vi "AB_Engine_CreateMissingVIsTree.vi"(10 "All VIs":T1[](array[typedef]), 11 "Missing VIs":T1[](array[typedef])) -> (3 "Missing VIs tree":variant)   [LabVIEW 2020]
uses:
  <vilib>/AppBuilder/Engine/AB_Engine_PathNode.ctl
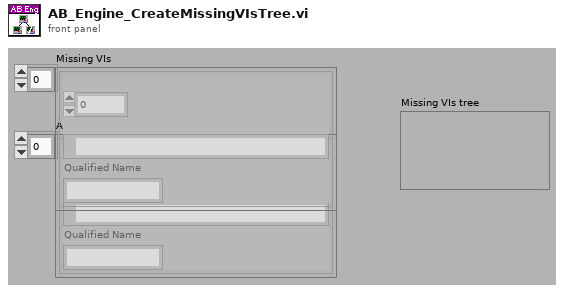
[diagram p1: front panel]
types:
  T1 = typedef "AB_Engine_PathNode.ctl" = cluster{"parent":i32, "path":path, "Qualified Name":string}
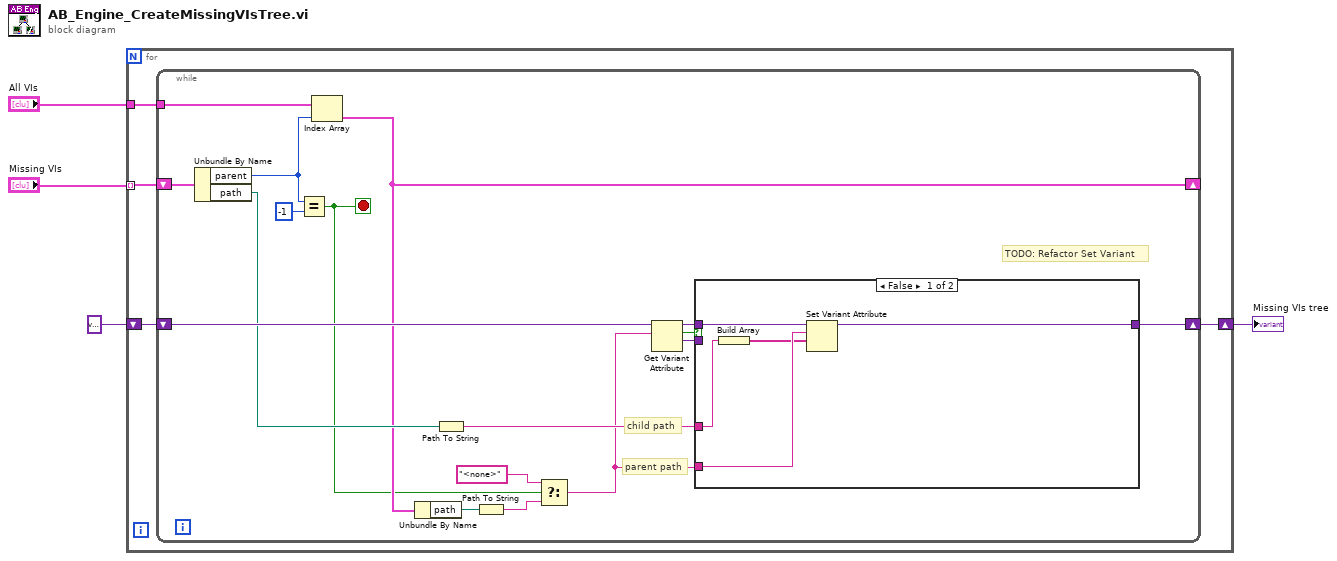
[diagram p0: block diagram]
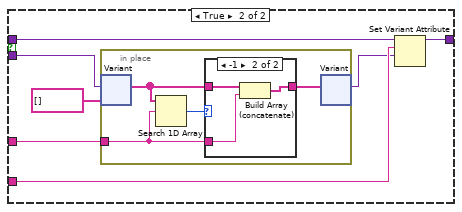
[diagram p2: hidden frame]
diagram:
  n1 = for {
    tunnel: "Missing VIs" -> [w7] mode=indexing
    tunnel: "All VIs" -> [w8]
    shift-right: [w5] -> w1
    shift-left: variant ("Node indices") -> [w6]
    n2 = while {
      tunnel: w8 -> [w25]
      shift-right: [w18] -> _
      shift-left: w7 -> [w20]
      shift-right: [w21] -> w5
      shift-left: w6 -> [w22]
      stop <- w11 stop-if-true
      # "TODO: Refactor Set Variant"
      # "parent path"
      # "child path"
      n3 = Unbundle By Name(w20) -> ("parent"=w24:i32, "path"=w19:path)
      n4 = Equal?(x=w24, y=-1) -> (x = y?=w11:bool)
      n5 = Index Array(array=w25, index=w24) -> (element=w18:T1)
      n6 = Unbundle By Name(w18) -> ("path"=w13:path)
      n7 = Path To String(path=w19) -> (string=w14:string)
      n8 = Path To String(path=w13) -> (string=w10:string)
      n9 = Select(t="<none>" ("f"), s=w11, f=w10) -> (s? t:f=w12:string)
      n10 = Get Variant Attribute(Variant=w22, name=w12) -> (duplicate Variant=w17:variant, found=w16:bool, value=w15:variant)  [unwired: 2 in, 1 out]
      n11 = case shown="False" w16 {
        tunnel: [w29 w37] -> w21
        tunnel: w17 -> [w30 w35]
        tunnel: w15 -> [_ w36]
        tunnel: w12 -> [w28 w34]
        tunnel: w14 -> [w27 w33]
        frame False {
          n12 = Build Array(w27) -> (w26:string[])
          n13 = Set Variant Attribute(Variant=w30, name=w28, value=w26) -> (Variant out=w29:variant)  [unwired: 1 in, 2 out]
        }
        frame True {
          n14 = in-place {
            in-place-border: w33 -> [w38]
            n15 = in-place-variant #1(w36, string[] []) -> (w40:string[])  [unwired: 1 out]
            n16 = Search 1D Array(1D array=w40, element=w38) -> (index of element=w39:i32)  [unwired: 1 in]
            n17 = case shown="-1" w39 {
              tunnel: [w42 w43] -> w41
              tunnel: w40 -> [w42 w44]
              tunnel: w38 -> [_ w45]
              frame Default {
              }
              frame -1 {
                n18 = Build Array (concatenate)(w44, w45) -> (w43:string[])
              }
            }
            n19 = in-place-variant #1(w41) -> (w31:variant)  [unwired: 1 out]
          }
          n20 = Set Variant Attribute(Variant=w35, name=w34, value=w31) -> (Variant out=w37:variant)  [unwired: 1 in, 2 out]
        }
      }
    }
  }
  "Missing VIs tree" <- w1
